vi "iFlex - Prepare for Acquisition.vi"() -> (3 "Open iFlex Global Shutter":variant)   [LabVIEW 2020]
uses:
  _Globals/Global Controls.vi
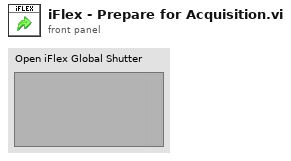
[diagram p1: front panel]
types:
  T1 = typedef "Tweezertron Ctrl Refs.ctl" = cluster{"LSM Settings":refnum<vi>, "iFlex Control":refnum<vi>, "PIFOC Settings":refnum<vi>, "PinSelector":refnum<vi>, "Manlight Controls":refnum<vi>, "Exp Params":refnum<vi>, "Image Thresholds":refnum<vi>, "RevFrame":refnum<vi>, "Spots":refnum<vi>}
  T2 = typedef "iFlex.ctl" = cluster{"561":dbl, "488":dbl, "Global Shutter":bool, "561 Shutter":bool}
  T3 = cluster{"notification":string, "Variant":variant}
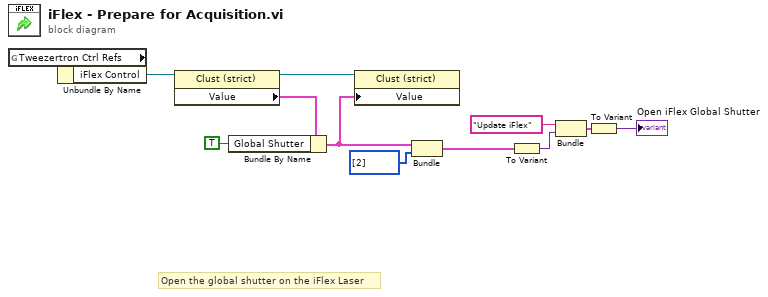
[diagram p0: block diagram]
diagram:
  # "Open the global shutter on the iFlex Laser"
  n1 = global read "Global Controls.vi" "Tweezertron Ctrl Refs"() -> (w8:T1)
  n2 = Unbundle By Name(w8) -> ("iFlex Control"=w7:refnum<vi>)
  n3 = property on="Property Node" class="Clust (strict)"(reference=w7) -> (reference out=w6:refnum<vi>, "Value"=w12:T2)  [unwired: 1 in, 1 out]
  n4 = Bundle By Name(cluster=w12, "Global Shutter"=TRUE) -> (w11:T2)
  n5 = property on="Property Node" class="Clust (strict)"(reference=w6, "Value"=w11) -> ()  [unwired: 1 in, 2 out]
  n6 = Bundle("Value"=w11, "appended array"=i32[] [2]) -> (w3:cluster{"Value":T2, "appended array":i32[]})  [unwired: 1 in]
  n7 = To Variant(anything=w3) -> (Variant=w2:variant)
  n8 = Bundle("notification"="Update iFlex", "Variant"=w2) -> (w4:T3)  [unwired: 1 in]
  n9 = To Variant(anything=w4) -> (Variant=→"Open iFlex Global Shutter":variant)
